vi "Parse.vi"(8 "Error In":errorcluster, 11 "reference in":refnum<class "2020_20.lvclass">) -> (0 "Error Out":errorcluster, 3 "reference out":refnum<class "2020_20.lvclass">)   [LabVIEW 2023, in "2020_20.lvclass"]
uses:
  2020_20.lvclass
  2020_20.lvclass/2020_20.ctl
  <userlib>/_OpenG.lib/string/string.llb/openg_string.lvlib
panel:
  out "Images":cluster{"Numeric":i32, "Array":bool[][]}[](array[cluster])
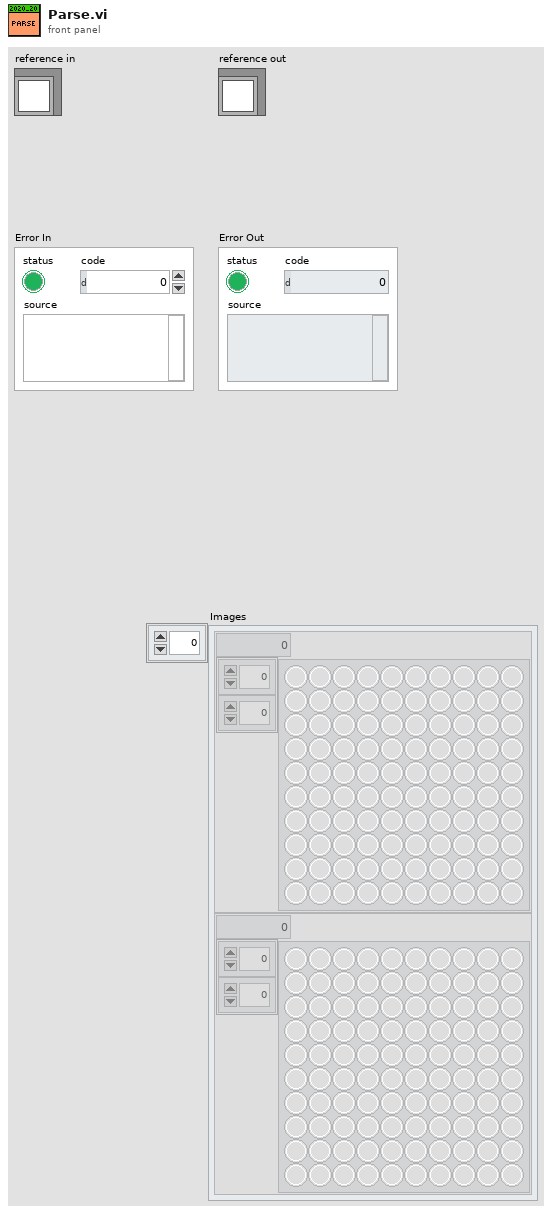
[diagram p1: front panel]
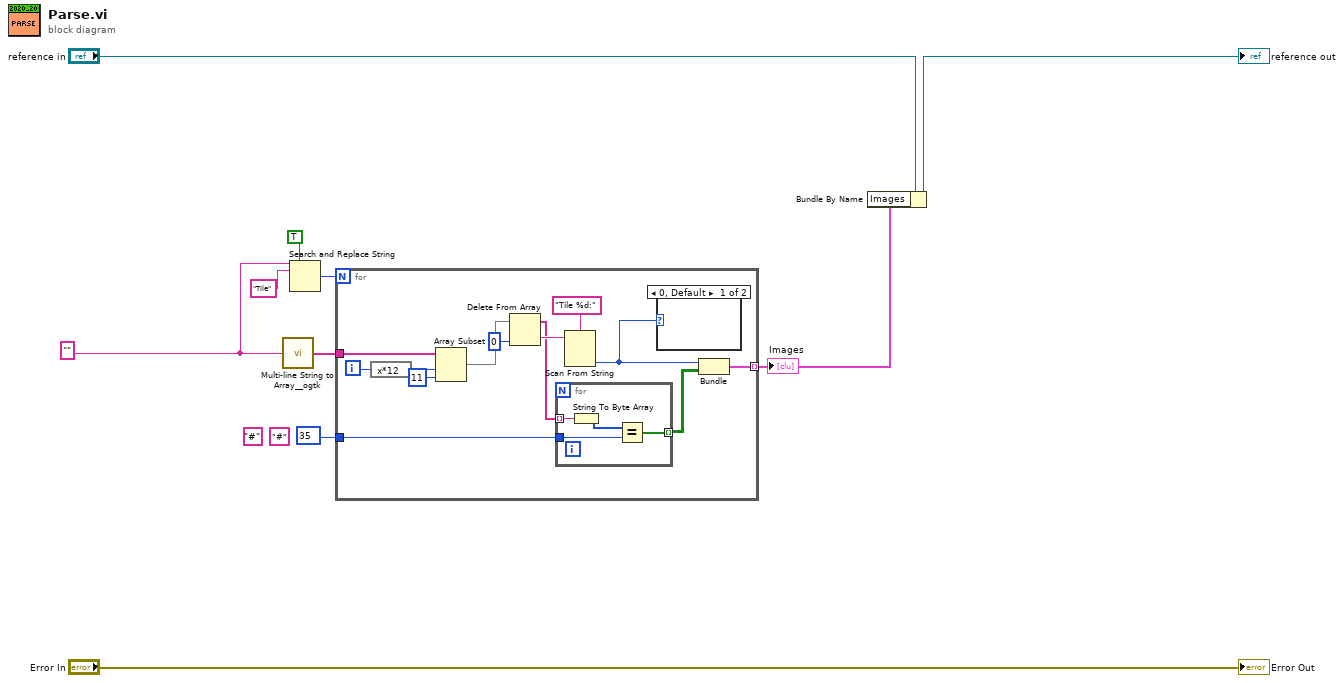
[diagram p0: block diagram]
diagram:
  (unwired) "#" ("search string")
  (unwired) "#" ("search string")
  w7 = "" ("PuzzleInput")
  n1 = call <userlib>:"Multi-line String to Array__ogtk.vi"("string"=w7) -> ("lines"=w3:string[])
  n2 = Search and Replace String(replace all?=TRUE ("replace all? (F)"), input string=w7, search string="Tile") -> (number of replacements=w4:i32)  [unwired: 5 in, 3 out]
  n3 = for {
    N: w4 -> [_]
    tunnel: w3 -> [w23]
    tunnel: 35 ("length") -> [w14]
    tunnel: [w12] -> w1 mode=indexing
    i -> [w22]
    n4 = expression code="x*12"(w22) -> (w21:i32)
    n5 = Array Subset(array=w23, index=w21, length=11) -> (w19:string[])
    n6 = Delete From Array(array=w19, index=0) -> (deleted portion=w17:string, array with subset deleted=w15:string[])  [unwired: 1 in]
    n7 = for {
      tunnel: w15 -> [w27] mode=indexing
      tunnel: w14 -> [w25]
      tunnel: [w24] -> w13 mode=indexing
      n8 = String To Byte Array(string=w27) -> (unsigned byte array=w26:u8[])
      n9 = Equal?(x=w26, y=w25) -> (x = y?=w24:bool[])
    }
    n10 = Scan From String(format string="Tile %d:", input string=w17) -> (output 1=w11:i32)  [unwired: 3 in, 3 out]
    n11 = case shown="0, Default" w11 {
      frame 0, Default {
      }
      frame 1.. {
      }
    }
    n12 = Bundle(w11, w13) -> (w12:cluster{i32, bool[][]})  [unwired: 1 in]
  }
  "Images" <- w1
  n13 = Bundle By Name(cluster="reference in", "Images"=w1) -> (→"reference out":refnum<class "2020_20.lvclass">)
  "Error Out" <- "Error In"
